vi "设置仪器参数命令解析.vi"(8 "error in (no error)":errorcluster caption="错误输入（无错误）", 11 "String输入":string) -> (0 "error out":errorcluster caption="错误输出", 3 "设置参数信息数组":string[][](array[string]))   [LabVIEW 2016, in "数据传输系统-05.lvlib"]
panel:
  out "大小":i32[](array[numeric])
  out "数组":string[](array[string])
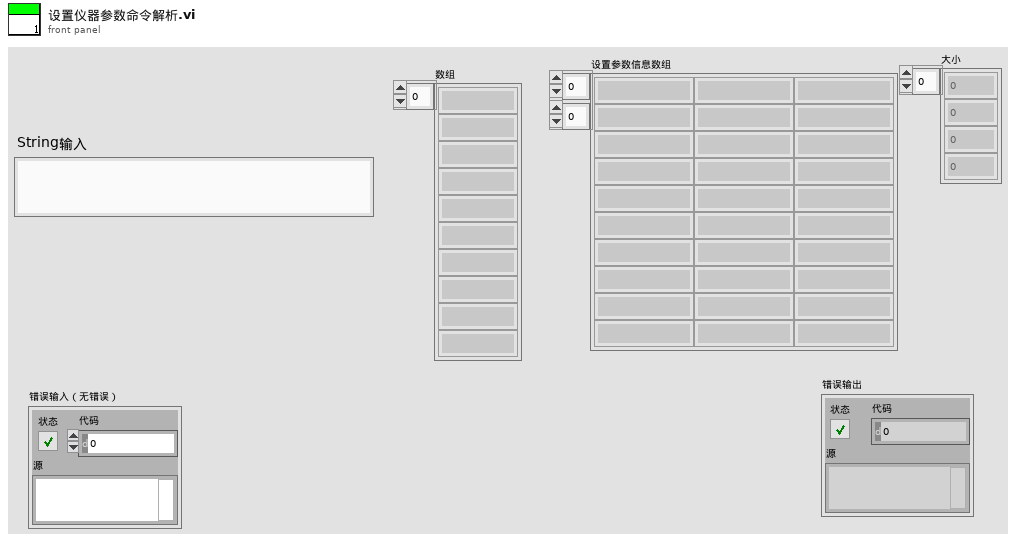
[diagram p1: front panel]
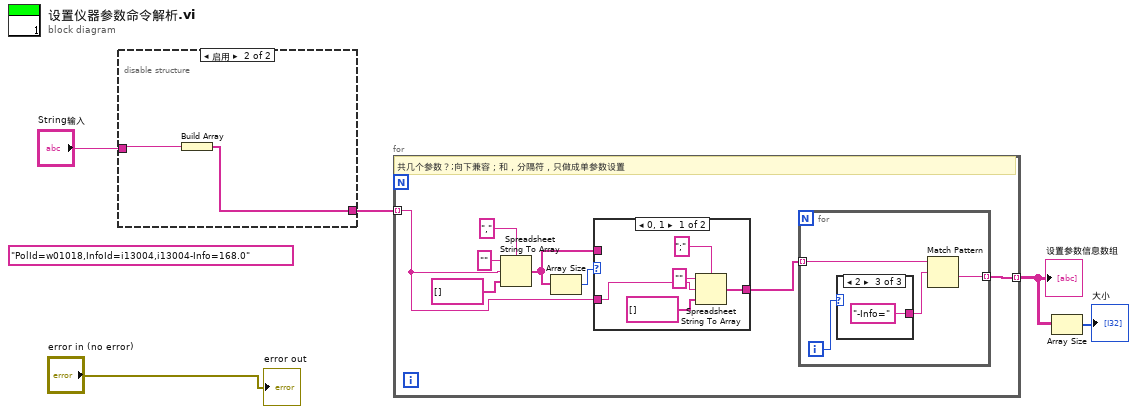
[diagram p0: block diagram]
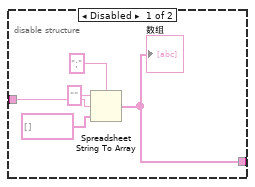
[diagram p2: hidden frame]
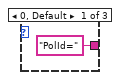
[diagram p4: hidden frame]
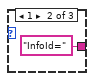
[diagram p5: hidden frame]
diagram:
  (unwired) "PolId=w01018,InfoId=i13004,i13004-Info=168.0"
  n1 = disable-structure shown="启用" {
    disable-tunnel: "String输入" -> [w8 w12]
    disable-tunnel: [w6 w11] -> w3
    frame Disabled {
      n2 = Spreadsheet String To Array(delimiter (Tab)=";" ("分隔符(Tab)"), format string="" ("格式字符串"), spreadsheet string=w8, array type (2D Dbl)=string[] []) -> (array=w6:string[])
      "数组" <- w6
    }
    frame Enabled {
      n3 = Build Array(w12) -> (w11:string[])
    }
  }
  n4 = for {
    tunnel: w3 -> [w15] mode=indexing
    tunnel: [w17] -> w1 mode=indexing
    # "共几个参数？;向下兼容；和，分隔符，只做成单参数设置"
    n5 = Spreadsheet String To Array(delimiter (Tab)="," ("分隔符(Tab)"), format string="" ("格式字符串"), spreadsheet string=w15, array type (2D Dbl)=string[] []) -> (array=w13:string[])
    n6 = Array Size(array=w13) -> (size(s)=w16:i32)
    n7 = case shown="0, 1" w16 {
      tunnel: w15 -> [w22 _]
      tunnel: [w21 w26] -> w14
      tunnel: w13 -> [_ w26]
      frame 0, 1 {
        n8 = Spreadsheet String To Array(delimiter (Tab)=";" ("分隔符(Tab)"), format string="" ("格式字符串"), spreadsheet string=w22, array type (2D Dbl)=string[] []) -> (array=w21:string[])
      }
      frame 2, Default {
      }
    }
    n9 = for {
      tunnel: w14 -> [w30] mode=indexing
      tunnel: [w27] -> w17 mode=indexing
      i -> [w29]
      n10 = case shown="2" w29 {
        tunnel: ["PolId=" "InfoId=" "-Info="] -> w28
        frame 0, Default {
        }
        frame 1 {
        }
        frame 2 {
        }
      }
      n11 = Match Pattern(string=w30, regular expression=w28) -> (after substring=w27:string)  [unwired: 1 in, 3 out]
    }
  }
  "设置参数信息数组" <- w1
  n12 = Array Size(array=w1) -> (size(s)=→"大小":i32[])
  "error out" <- "error in (no error)"
